vi "PositiveSpectralValues (SubVI).vi"(10 "Size of Positive Half of FFT":dbl, 11 "Scaled Full Length FFT":dbl[](array[numeric])) -> (3 "Positve Half of FFT with 0Hz and Nyquist":dbl[](array[numeric]))   [LabVIEW 2015]
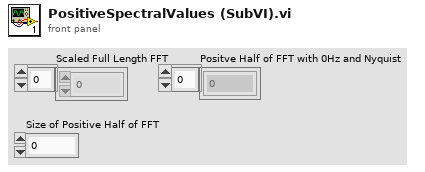
[diagram p1: front panel]
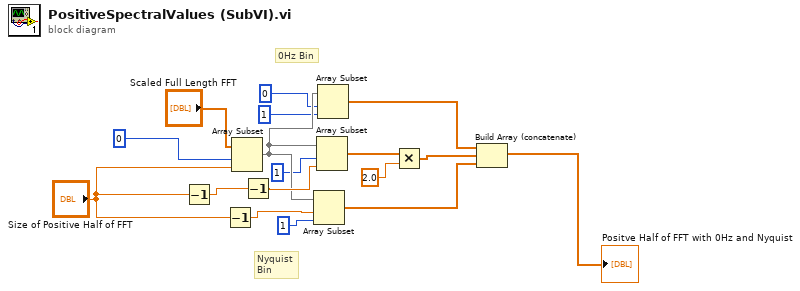
[diagram p0: block diagram]
diagram:
  # "Nyquist Bin"
  # "0Hz Bin"
  n1 = Decrement(x="Size of Positive Half of FFT") -> (x-1=w3:dbl)
  n2 = Decrement(x="Size of Positive Half of FFT") -> (x-1=w1:dbl)
  n3 = Array Subset(array="Scaled Full Length FFT", index=0, length="Size of Positive Half of FFT") -> (w12:dbl[])
  n4 = Decrement(x=w3) -> (x-1=w16:dbl)
  n5 = Array Subset(array=w12, index=w1, length=1) -> (w11:dbl[])
  n6 = Array Subset(array=w12, index=1, length=w16) -> (w13:dbl[])
  n7 = Array Subset(array=w12, index=0, length=1) -> (w10:dbl[])
  n8 = Multiply(x=w13, y=2.0) -> (x*y=w15:dbl[])
  n9 = Build Array (concatenate)(w10, w15, w11) -> (→"Positve Half of FFT with 0Hz and Nyquist":dbl[])
